vi "GET STOP(WithError).vi"(9 "error in (no error)":errorcluster) -> (8 "Stop":bool, 10 "error out":errorcluster)   [LabVIEW 2012, in "GlobalStop(dev).lvlib"]
uses:
  GlobalStop(dev).lvlib
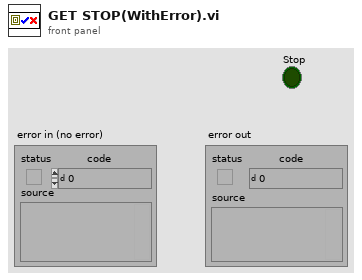
[diagram p1: front panel]
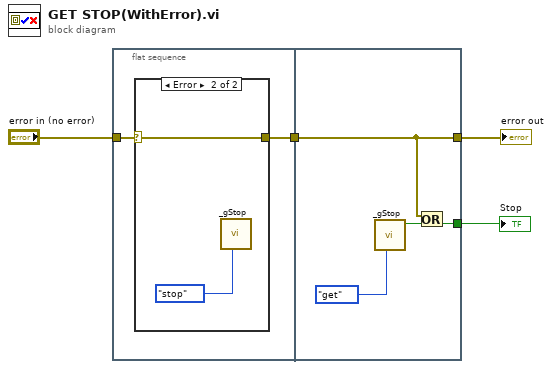
[diagram p0: block diagram]
diagram:
  n1 = flat-sequence {
    tunnel: "error in (no error)" -> [w6]
    tunnel: [w5] -> w1
    tunnel: [w11] -> w4
    tunnel: [w10] -> w2
    tunnel: w1 -> [w10]
    frame #0 {
      n2 = case shown="Error" w6 {
        selector: w6 -> [w7 w8]
        tunnel: [w7 w8] -> w5
        frame No Error {
        }
        frame Error {
          n3 = call "_gStop.vi"("op"=enum16{"reset", "get", "stop"}."stop") -> ()  [unwired: 10 in, 1 out]
        }
      }
    }
    frame #1 {
      n4 = call "_gStop.vi"("op"=enum16{"reset", "get", "stop"}."get") -> ("Boolean"=w12:bool)  [unwired: 10 in]
      n5 = Or(x=w10, y=w12) -> (x .or. y?=w11:bool)
    }
  }
  "error out" <- w2
  "Stop" <- w4
